vi "GetChannelInfo.vi"(8 "error in (no error)":errorcluster, 10 "Channel":u8, 11 "ID":i32) -> (0 "error out":errorcluster, 2 "Channel information":T1 {"NbAmp" min=5 max=7; "LcBoard" min=5 max=7; "AmpCode" min=5 max=7}, 3 "ID Out":i32)   [LabVIEW 2022 SP3, in "EClib functions.lvlib"]
doc: "This VI supplies information on the selected channel."
uses:
  EClib functions.lvlib
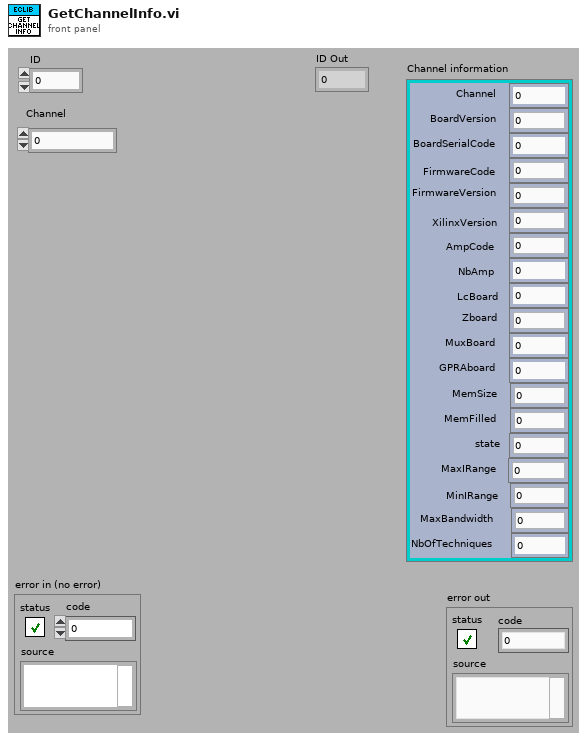
[diagram p1: front panel]
types:
  T1 = cluster{"Channel":i32, "BoardVersion":i32, "BoardSerialCode":i32, "FirmwareCode":i32, "FirmwareVersion":i32, "XilinxVersion":i32, "AmpCode":i32, "NbAmp":i32, "LcBoard":i32, "Zboard":i32, "MuxBoard":i32, "GPRAboard":i32, "MemSize":i32, "MemFilled":i32, "state":i32, "MaxIRange":i32, "MinIRange":i32, "MaxBandwidth":i32, "NbOfTechniques":i32}
  T2 = cluster{"Channel":i32, "BoardVersion":i32, "BoardSerialCode":i32, "FirmwareCode":i32, "FirmwareVersion":i32, "XilinxVersion":i32, "AmpCode":i32, "NbAmp":i32, "LcBoard":i32, "Zboard":i32, "MuxBoard":i32, "GPRAboard":i32, "MemSize":i32, "MemFilled":i32, "state":i32, "MaxeRange":i32, "MinRange":i32, "MaxBandwidth":i32, "NbOfTechniques":i32}
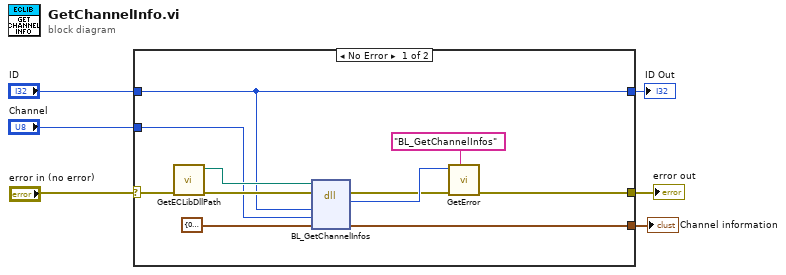
[diagram p0: block diagram]
diagram:
  n1 = case shown="No Error" "error in (no error)" {
    selector: "error in (no error)" -> [w10 w19]
    tunnel: [w15 w19] -> w5
    tunnel: [w13 _] -> w4
    tunnel: "Channel" -> [w8 _]
    tunnel: "ID" -> [w7 w18]
    tunnel: [w7 w18] -> w1
    frame No Error {
      n2 = call "GetECLibDllPath.vi"("error in (no error)"=w10) -> ("error out"=w9:errorcluster, "ECLibDLLPath"=w17:path)  [unwired: 9 in]
      n3 = dll-call lib="?" fn="BL_GetChannelInfos"(path in=w17, error in=w9, "arg1"=w7, "arg2"=w8, "arg3"=T2 {"Channel"=0, "BoardVersion"=0, "BoardSerialCode"=0, "FirmwareCode"=0, "FirmwareVersion"=0, "XilinxVersion"=0, "AmpCode"=0, "NbAmp"=0, "LcBoard"=0, "Zboard"=0, "MuxBoard"=0, "GPRAboard"=0, "MemSize"=0, "MemFilled"=0, "state"=0, "MaxeRange"=0, "MinRange"=0, "MaxBandwidth"=0, "NbOfTechniques"=0} ("Channel information")) -> (error out=w12:errorcluster, "return type"=w14:i32, "arg3"=w13:T2)  [unwired: 3 in, 1 out]
      n4 = call "GetError.vi"("DLLFunction"="BL_GetChannelInfos", "error in"=w12, "code"=w14) -> ("error out"=w15:errorcluster)  [unwired: 8 in]
    }
    frame Error {
    }
  }
  "error out" <- w5
  "Channel information" <- w4
  "ID Out" <- w1
